vi "Set Output Data Bit.vi"(0 "BIT Set/Clear":bool, 5 "index":i32=1, 7 "ChannelList":string="201:201", 9 "instrument handle":refnum<k15>="USB0::0x2A8D::0x5001::MY58000421::INSTR", 11 "error in (no error)":errorcluster {"code" format="%.0x"}) -> (4 "error out":errorcluster {"code" format="%.0x"})   [LabVIEW 2016]
uses:
  <instrlib>/Keysight DAQ970/Keysight DAQ970.lvlib
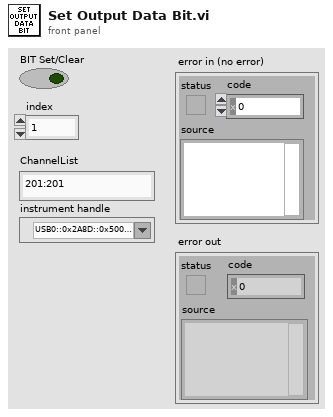
[diagram p1: front panel]
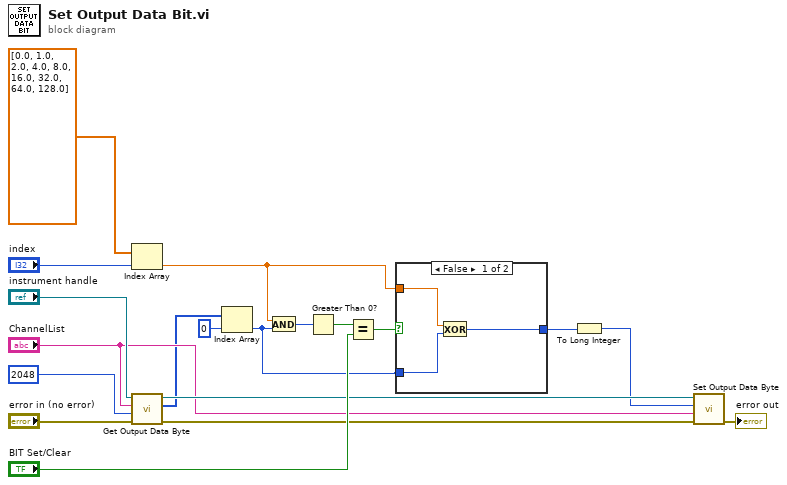
[diagram p0: block diagram]
diagram:
  n1 = Index Array(array=dbl[] [0.0, 1.0, 2.0, 4.0, 8.0, 16.0, 32.0, 64.0, 128.0], index="index") -> (element=w2:dbl)
  n2 = call <instrlib>:"Get Output Data Byte.vi"("error in (no error)"="error in (no error)", "ValBufferSize"=2048, "ChannelList"="ChannelList", "instrument handle"="instrument handle") -> ("error out"=w14:errorcluster, "Val"=w4:i32[], "instrument handle out"=w13:refnum<k15>)  [unwired: 4 in, 1 out]
  n3 = Index Array(array=w4, index=0) -> (element=w3:i32)
  n4 = And(x=w2, y=w3) -> (x .and. y?=w7:i32)
  n5 = Greater Than 0?(x=w7) -> (x > 0?=w6:bool)
  n6 = Equal?(x=w6, y="BIT Set/Clear") -> (x = y?=w1:bool)
  n7 = case shown="False" w1 {
    tunnel: w3 -> [w20 w23]
    tunnel: [w22 w23] -> w10
    tunnel: w2 -> [w21 _]
    frame False {
      n8 = Exclusive Or(1:w20, 2:w21) -> (0:w22:i32)
    }
    frame True {
    }
  }
  n9 = To Long Integer(number=w10) -> (32bit integer=w9:i32)
  n10 = call <instrlib>:"Set Output Data Byte.vi"("error in (no error)"=w14, "ChannelList"="ChannelList", "Data"=w9, "instrument handle"=w13) -> ("error out"=→"error out":errorcluster)  [unwired: 6 in, 1 out]
